vi "GPS.vi"() -> (0 "Waveform Chart":dbl(graph)=-87.32227227105035, 1 "Waveform Chart 2":dbl(graph)=39.483871392144096)   [LabVIEW 2011]
uses:
  <instrlib>/NavCom SF-2050/NavCom SF-2050.lvlib
panel:
  in  "stop":bool=TRUE
  out "Satellites Used":i32[](array[numeric])=[6, 11, 15, 21, 24, 27, 30, 31]
  out "Velocity, Correction & SET":T1={"Velocity North"=-178.0, "Velocity East"=-32.0, "Velocity Up"=-14.0, "Ellipsoidal Height"=128.47265625, "GDOP"=4.3, "PDOP"=3.4, "HDOP"=1.4, "VDOP"=3.1, "TDOP"=2.5, "Horizontal Figure of Merit"=255, "Time Figure of Merit"=216, "Max dGPS Age"=0.0, "Extended Navigation Mode"=0, "Antenna Height Adjustment "=0.0, "SET North"=0, "SET East"=0, "SET Up"=0} {"Extended Navigation Mode" items=["Non Differential"=0, "Code (RTCM Type 1 & 9)"=1, "Code, Single Frequency (WAAS)"=2, "Code, Dual Frequency (WAAS)"=3, "Code, Single Frequency (WCT)"=4, "Code/RCP, Dual Frequency (WCT)"=5, "Code, Single Frequency (RTG)"=6, "Code (RTCM Type 1 & 9) Dual Frequency"=10, "Code/RCP, Dual Frequency (RTG)"=11, "Code, Single Frequency (NCT-RTK)"=12, "Code, Single Frequency (RTCM 18 & 19)"=13, "Code, Single Frequency (RTCM 21 & 22)"=14, "Code, Single Frequency (CMR)"=15, "Code, Dual Frequency (NCT-RTK)"=16, "Code, Dual Frequency (RTCM 18 & 19)"=17, "Code, Dual Frequency (RTCM 20 & 21)"=18, "Code, Dual Frequency (CMR)"=19, "RTK (NCT-RTK)"=20, "RTK (RTCM 18 & 19)"=21, "RTK (RTCM 20 & 21)"=22, "RTK (CMR)"=23, "Code, Single Frequency with SET (RTG)"=24, "Code/RCP, Dual Frequency with SET (RTG)"=25, "RTK Extend"=26]}
  out "Altitude":dbl=165.5244140625
  out "Longitude":dbl=-87.32227227105035
  out "Latitude":dbl=39.483871392144096
  out "Time":cluster{"GPS Week":u16, "GPS Time of Week":sgl}={"GPS Week"=1679, "GPS Time of Week"=264981.6} {"GPS Time of Week" format="%.3f"}
  out "error out":errorcluster
  in  "Serial Configuration":cluster{"Baud Rate":u32, "Parity":u16}={"Baud Rate"=115200, "Parity"=0} {"Parity" items=["None", "Odd", "Even", "Mark", "Space"]; "Baud Rate" items=["1200"=1200, "2400"=2400, "4800"=4800, "9600"=9600, "19200"=19200, "38400"=38400, "57600"=57600, "115200"=115200]}
  in  "VISA resource name":refnum<visa-resource-name>="COM17"
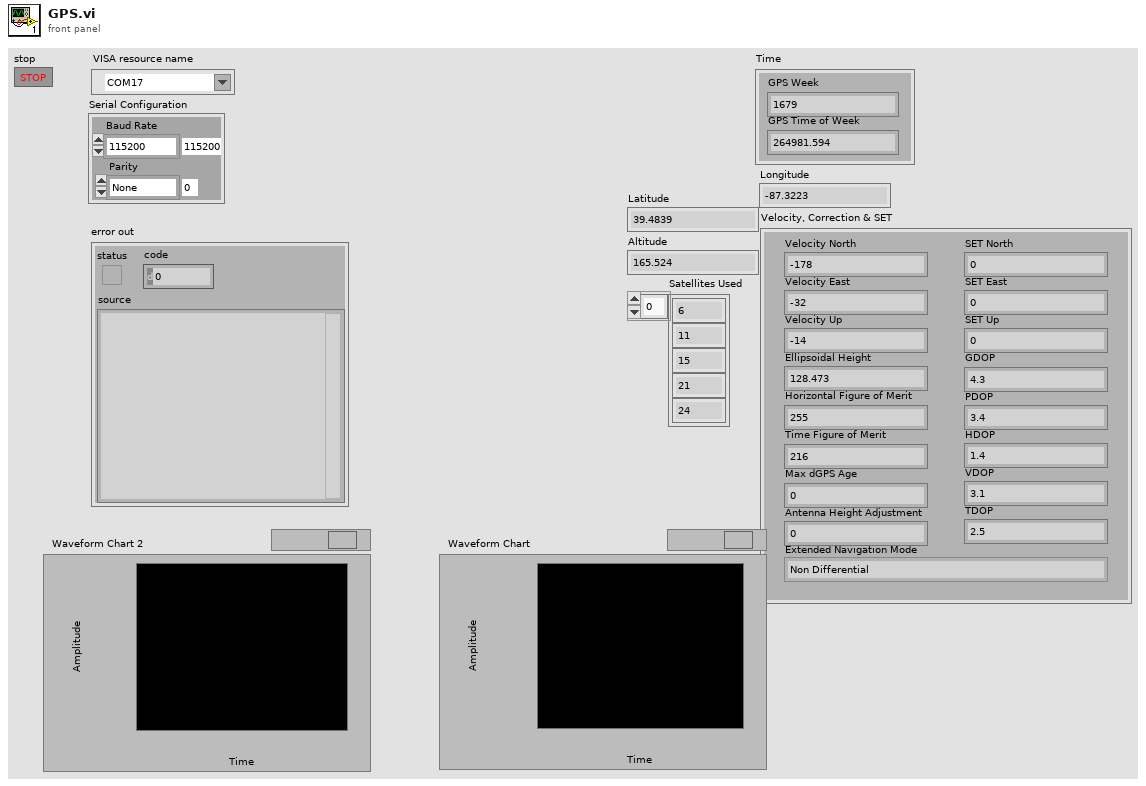
[diagram p1: front panel]
types:
  T1 = cluster{"Velocity North":dbl, "Velocity East":dbl, "Velocity Up":dbl, "Ellipsoidal Height":dbl, "GDOP":sgl, "PDOP":sgl, "HDOP":sgl, "VDOP":sgl, "TDOP":sgl, "Horizontal Figure of Merit":u8, "Time Figure of Merit":u8, "Max dGPS Age":sgl, "Extended Navigation Mode":u8, "Antenna Height Adjustment ":dbl, "SET North":i32, "SET East":i32, "SET Up":i32}
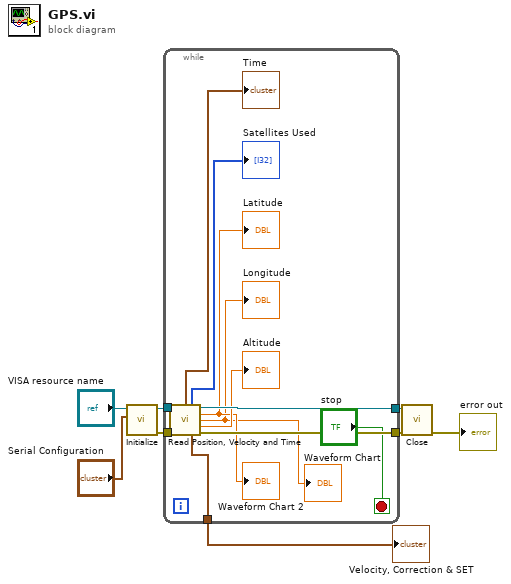
[diagram p0: block diagram]
diagram:
  n1 = call <instrlib>:"Initialize.vi"("Serial Configuration"="Serial Configuration", "VISA resource name"="VISA resource name") -> ("error out"=w4:errorcluster, "VISA resource name out"=w8:refnum<visa-resource-name>)  [unwired: 8 in]
  n2 = while {
    tunnel: w8 -> [w19]
    tunnel: [w18] -> w7
    tunnel: w4 -> [w17]
    tunnel: [w16] -> w3
    tunnel: [w13] -> w1
    stop <- "stop" stop-if-true
    n3 = call <instrlib>:"Read Position, Velocity and Time.vi"("VISA resource name"=w19, "error in (no error)"=w17) -> ("Time"=→"Time":cluster{"GPS Week":u16, "GPS Time of Week":sgl}, "Satellites Used"=→"Satellites Used":i32[], "VISA resource name out"=w18:refnum<visa-resource-name>, "Latitude"=→"Latitude" →"Waveform Chart 2":dbl, "Longitude"=→"Longitude" →"Waveform Chart":dbl, "Altitude"=→"Altitude":dbl, "Velocity, Correction & SET"=w13:T1, "error out"=w16:errorcluster)  [unwired: 6 in]
  }
  "Velocity, Correction & SET" <- w1
  n4 = call <instrlib>:"Close.vi"("error in (no error)"=w3, "VISA resource name"=w7) -> ("error out"=→"error out":errorcluster)  [unwired: 9 in]
